vi "centered_ring_bounds.vi"(3 "radius R":dbl, 5 "Image":T1) -> (1 "Bounding Rectangle":T2)   [LabVIEW 2011]
doc: "Creates a bounding rectangle for a overlay ring of radius R centerd in the image."
uses:
  <vilib>/vision/Image Controls.llb/IMAQ Image.ctl
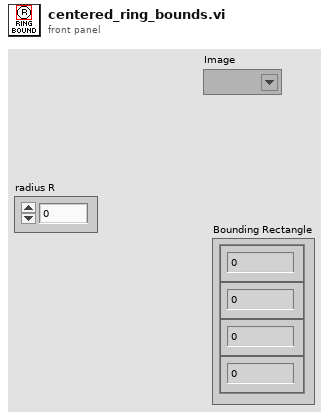
[diagram p1: front panel]
types:
  T1 = typedef "IMAQ Image.ctl" = refnum<image>
  T2 = cluster{"Numeric Control":dbl, "Numeric Control":dbl, "Numeric Control":dbl, "Numeric Control":dbl}
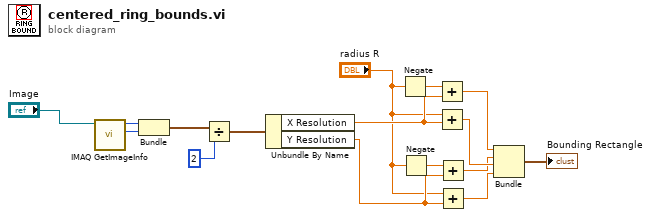
[diagram p0: block diagram]
diagram:
  n1 = call "IMAQ GetImageInfo"("Image"="Image") -> ("Y Resolution"=w3:i32, "X Resolution"=w4:i32)  [unwired: 3 in, 6 out]
  n2 = Bundle("X Resolution"=w4, "Y Resolution"=w3) -> (w2:cluster{"X Resolution":i32, "Y Resolution":i32})  [unwired: 1 in]
  n3 = Divide(x=w2, y=2 ("y height(Px)")) -> (x/y=w5:cluster{"X Resolution":dbl, "Y Resolution":dbl})
  n4 = Unbundle By Name(w5) -> ("X Resolution"=w14:dbl, "Y Resolution"=w10:dbl)
  n5 = Negate(x="radius R") -> (-x=w15:dbl)
  n6 = Negate(x="radius R") -> (-x=w11:dbl)
  n7 = Add(x=w15, y=w14) -> (x+y=w13:dbl)
  n8 = Add(x="radius R", y=w14) -> (x+y=w12:dbl)
  n9 = Add(x=w11, y=w10) -> (x+y=w8:dbl)
  n10 = Add(x="radius R", y=w10) -> (x+y=w7:dbl)
  n11 = Bundle(w13, w8, w12, w7) -> (→"Bounding Rectangle":cluster{dbl, dbl, dbl, dbl})  [unwired: 1 in]
